vi "Init Tx Data.vi"(7 "Data Access in":refnum<class "Data Access Engine.lvclass">, 8 "error in (no error)":errorcluster, 11 "Parameters":variant) -> (0 "error out":errorcluster, 3 "Tx Loop Data":T1, 5 "Data Access out":refnum<class "Data Access Engine.lvclass">)   [LabVIEW 2016, in "UDP-Custom-Device Engine.lvlib"]
uses:
  UDP-Custom-Device Engine.lvlib
  <vilib>/NI/NIVS Inline Async API/_Data Access Engine/Data Access Engine/Data Access Engine.lvclass
  Tx Loop Data.ctl
  <vilib>/NI Veristand/VeriStand Data/Library/Byte Buffer/Byte Buffer.lvclass
  <vilib>/NI/NIVS Inline Async API/_Data Access Engine/Data Access Engine/Types/Read.DVR.ctl
  <vilib>/NI/NIVS Inline Async API/_Data Access Engine/Access Type Classes/Read/Read.lvclass
  <vilib>/NI Veristand/VeriStand Data/Library/Typedefs/Typedefs.Data Types.ctl
  Data Conversion Config.ctl
  <vilib>/NI Veristand/VeriStand Data/Library/Byte Buffer/Byte Buffer.Mapping.ctl
  Shared/Header Details.ctl
  Shared/Tx.PacketInfo.ctl
  System Explorer/Types/Channel Data Type.ctl
  <vilib>/NI/NIVS Inline Async API/_Data Access Engine/Data Access Engine/Methods/Read.Lookup.vi
  Shared/UDP-Custom-Device Shared.lvlib
  <vilib>/NI Veristand/VeriStand Data/Library/VeriStand Data.lvlib
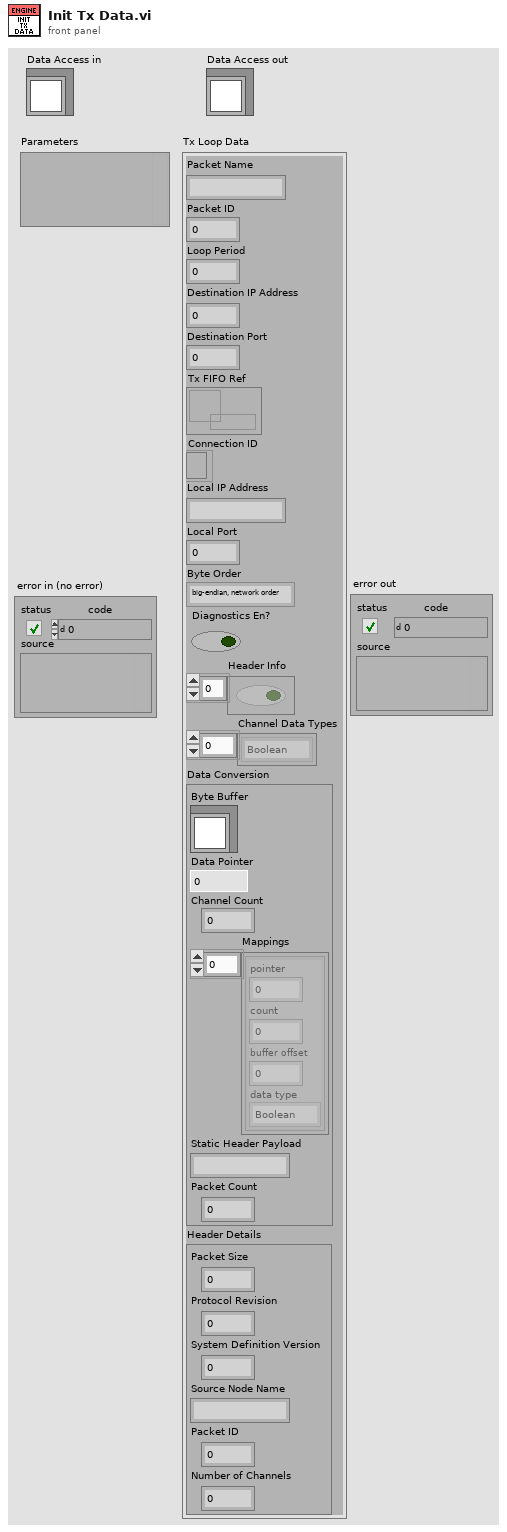
[diagram p1: front panel]
types:
  T1 = typedef "UDP-Custom-Device Engine.lvlib/Tx Loop Data.ctl" = cluster{"Packet Name":string, "Packet ID":i32, "Loop Period":u32, "Destination IP Address":u32, "Destination Port":u16, "Tx FIFO Ref":T2, "Connection ID":refnum<k16>, "Local IP Address":string, "Local Port":i32, "Byte Order":enum16{"big-endian, network order", "native, host order", "little-endian"}, "Diagnostics En?":bool, "Header Info":bool[], "Channel Data Types":T3[], "Data Conversion":T4, "Header Details":T6}
  T2 = typedef "Data Access Engine.lvlib/Data Access Engine.lvclass/Read.DVR.ctl" = refnum<data-value>
  T3 = typedef "VeriStand Data.lvlib/Typedefs.Data Types.ctl" = enum16{"Boolean", "Single", "Double", "I8", "I16", "I32", "I64", "U8", "U16", "U32", "U64"}
  T4 = typedef "UDP-Custom-Device Engine.lvlib/Data Conversion Config.ctl" = cluster{"Byte Buffer":refnum<class "Byte Buffer.lvclass">, "Data Pointer":u64, "Channel Count":i32, "Mappings":T5[], "Static Header Payload":string, "Packet Count":dbl}
  T5 = typedef "VeriStand Data.lvlib/Byte Buffer.lvclass/Byte Buffer.Mapping.ctl" = cluster{"pointer":u64, "count":i32, "buffer offset":i32, "data type":T3}
  T6 = typedef "UDP-Custom-Device Shared.lvlib/Header Details.ctl" = cluster{"Packet Size":u16, "Protocol Revision":u8, "System Definition Version":u16, "Source Node Name":string, "Packet ID":u32, "Number of Channels":u32}
  T7 = typedef "UDP-Custom-Device Shared.lvlib/Tx.PacketInfo.ctl" = cluster{"Packet Name":string, "Packet ID":i32, "Decimation":i32, "Destination IP Address":string, "Destination Port":i32, "Local IP Address":string, "Local Port":i32, "Endianness":u16, "Diagnostics En?":bool, "Header Info":bool[], "PCL Period":u32, "Channel Data Types":T8[]}
  T8 = typedef "UDP-Custom-Device Shared.lvlib/Channel Data Type.ctl" = enum16{"Boolean", "Single"}
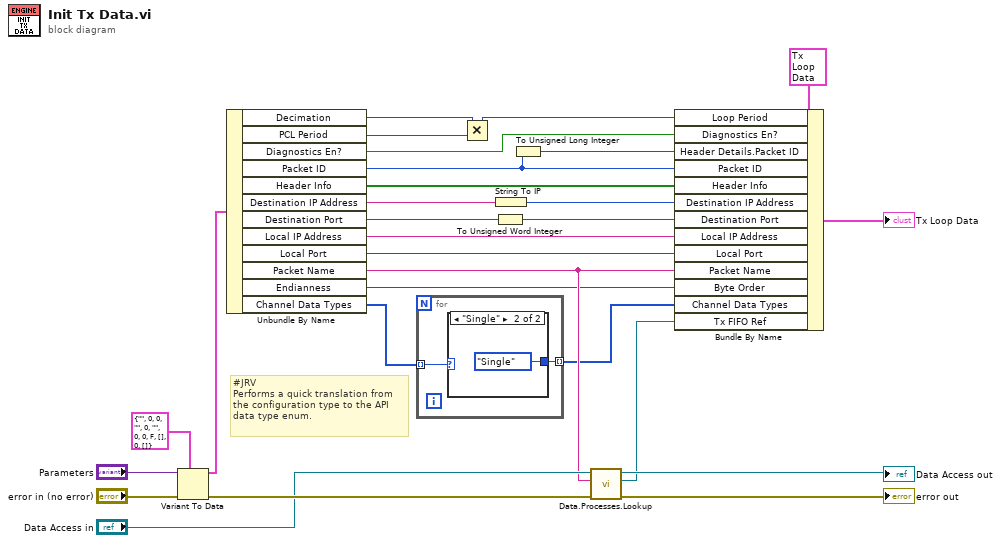
[diagram p0: block diagram]
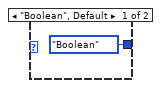
[diagram p2: hidden frame]
diagram:
  # "#JRV\nPerforms a quick translation from\nthe configuration type to the API\ndata type enum."
  n1 = Variant To Data(error in="error in (no error)", type=T7 {"Packet Name"="", "Packet ID"=0, "Decimation"=0, "Destination IP Address"="", "Destination Port"=0, "Local IP Address"="", "Local Port"=0, "Endianness"=0, "Diagnostics En?"=FALSE, "Header Info"=[], "PCL Period"=0, "Channel Data Types"=[]} ("Packet Info"), Variant="Parameters") -> (data=w26:T7, error out=w25:errorcluster)
  n2 = Unbundle By Name(w26) -> ("Decimation"=w10:i32, "PCL Period"=w11:u32, "Diagnostics En?"=w13:bool, "Packet ID"=w2:i32, "Header Info"=w12:bool[], "Destination IP Address"=w4:string, "Destination Port"=w6:i32, "Local IP Address"=w17:string, "Local Port"=w16:i32, "Packet Name"=w18:string, "Endianness"=w14:u16, "Channel Data Types"=w8:T8[])
  n3 = for {
    tunnel: w8 -> [w30] mode=indexing
    tunnel: [w29] -> w7 mode=indexing
    n4 = case shown="\"Single\"" w30 {
      tunnel: [Typedefs.Data_Types."Boolean" ("data type") Typedefs.Data_Types."Single" ("data type")] -> w29
      frame "Boolean", Default {
      }
      frame "Single" {
      }
    }
  }
  n5 = Multiply(x=w10, y=w11) -> (x*y=w9:u32)
  n6 = To Unsigned Word Integer(number=w6) -> (unsigned 16bit integer=w5:u16)
  n7 = String To IP(1:w4) -> (0:w3:u32)
  n8 = To Unsigned Long Integer(number=w2) -> (unsigned 32bit integer=w1:u32)
  n9 = call-poly <vilib>:"Data.Processes.Lookup.vi"("error in (no error)"=w25, "Name"=w18, "Data Access API in"="Data Access in") -> ("error out"=→"error out":errorcluster, "Ref"=w15:T2, "Data Access API out"=→"Data Access out":refnum<class "Data Access Engine.lvclass">)  [unwired: 5 in, 1 out]
  n10 = Bundle By Name(cluster=T1 {"Packet Name"="", "Packet ID"=0, "Loop Period"=0, "Destination IP Address"=0, "Destination Port"=0, "Tx FIFO Ref"=refnum, "Connection ID"=refnum, "Local IP Address"="", "Local Port"=0, "Byte Order"=enum."big-endian, network order", "Diagnostics En?"=FALSE, "Header Info"=[], "Channel Data Types"=[], "Data Conversion"={"Byte Buffer"=refnum, "Data Pointer"=0, "Channel Count"=0, "Mappings"=[], "Static Header Payload"="", "Packet Count"=0.0}, "Header Details"={"Packet Size"=0, "Protocol Revision"=0, "System Definition Version"=0, "Source Node Name"="", "Packet ID"=0, "Number of Channels"=0}} ("Tx Loop Data"), "Loop Period"=w9, "Diagnostics En?"=w13, "Header Details.Packet ID"=w1, "Packet ID"=w2, "Header Info"=w12, "Destination IP Address"=w3, "Destination Port"=w5, "Local IP Address"=w17, "Local Port"=w16, "Packet Name"=w18, "Byte Order"=w14, "Channel Data Types"=w7, "Tx FIFO Ref"=w15) -> (→"Tx Loop Data":T1)
